vi "Read Required Digits of Precision.vi"(11 "Floating Point in":refnum<class "Floating Point.lvclass">) -> (2 "Required Digits of Precision":u8=6)   [LabVIEW 2018, in "Floating Point.lvclass"]
uses:
  Floating Point.lvclass
  Floating Point.lvclass/Floating Point.ctl
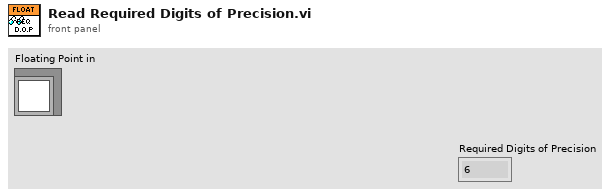
[diagram p1: front panel]
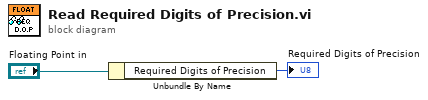
[diagram p0: block diagram]
diagram:
  n1 = Unbundle By Name("Floating Point in") -> ("Required Digits of Precision"=→"Required Digits of Precision":u8)
